vi "MemoryMapMain.vi"(8 "error in (no error)":errorcluster, 11 "MemoryMap in":refnum<class "MemoryMap.lvclass">) -> (3 "MemoryMap out":refnum<class "MemoryMap.lvclass">)   [LabVIEW 2020, in "Sgraph_lib_V1.lvlib" / "MemoryMap.lvclass"]
uses:
  MemoryMap.lvclass
  Gserver/controls/Typedef_Gviewer-Query.ctl
  Gserver/controls/Typedef_QueryType.ctl
  Common/controls/MeMapInfo.ctl
  Common/controls/MMap_element.ctl
  <vilib>/Utility/miscctls.llb/LVPoint32TypeDef.ctl
  Builds/Sgraph_lib_V1.lvlib
  Gserver/Gserver.lvclass
panel:
  in  "Layer":i32 min=0 max=6
  out "Graph 3":cluster{"Array":dbl[]}[](graph)
  out "Graph 2":cluster{"Array":dbl[]}[](graph)
  out "Graph 1":cluster{"Array":dbl[]}[](graph)
  out "37x37":picture
  in  "Gserver-Queue":refnum<queue>
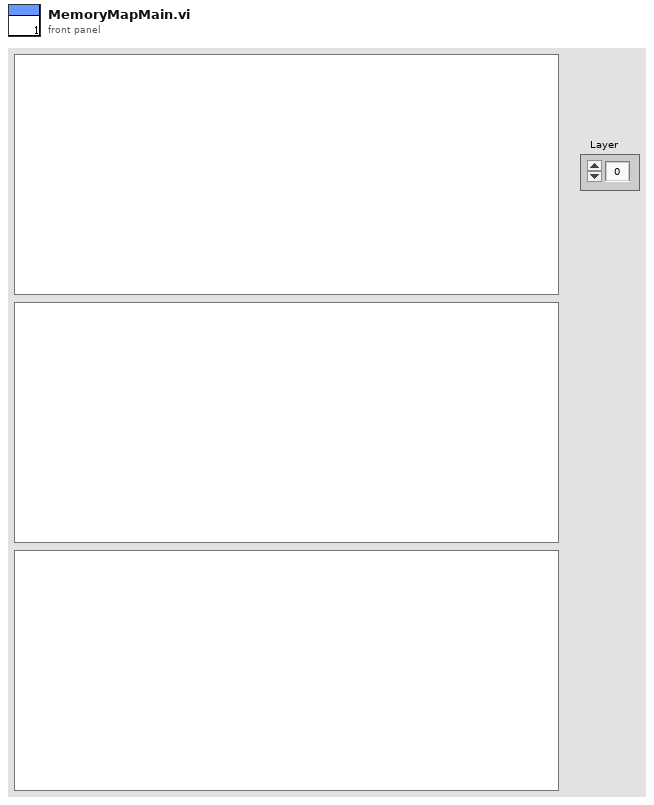
[diagram p1: front panel]
types:
  T1 = typedef "Sgraph_lib_V1.lvlib/MeMapInfo.ctl" = cluster{"MemLayer":T2[]}
  T2 = typedef "Sgraph_lib_V1.lvlib/MMap_element.ctl" = cluster{"Name":string, "Length":i32, "Pointer":i32, "Tbegin":dbl, "Tend":dbl, "Tmin":dbl, "Tmax":dbl, "Tpnt-1":dbl, "Tpnt":dbl, "Tpnt+1":dbl, "Array":dbl[]}
  T3 = typedef "LVBoundsTypeDef.ctl" = cluster{"Width":u32, "Height":u32}
  T4 = typedef "Sgraph_lib_V1.lvlib/Gserver.lvclass/Typedef_QueryType.ctl" = enum16{"Subscribe", "DataRequest", "RequestAllTags", "RequestIniPath", "FAMMstarted", "SetClientOptions", "GviewerUpdate", "OpenNewGraph", "CloseClient", "CloseAllClients", "Close Gserver", "OpenMemoryMap", "MeMapDataRequest", "MeMapDataResponse", "OpenDBeditor", "CheckDBeditorRunning", "StoppedDBeditor", "SaveDB_TAGpropRecord", "ConfirmDB_TAGpropSave"}
  T5 = typedef "Sgraph_lib_V1.lvlib/Gserver.lvclass/Typedef_Gviewer-Query.ctl" = cluster{"Query_type":T4, "data":variant, "Source":string, "Time Stamp":timestamp}
  T6 = cluster{"horizontal":enum16{"left", "center", "right"}, "vertical":enum16{"top", "center", "bottom"}}
  T7 = typedef "LVPoint32TypeDef.ctl" = cluster{"Horizontal":i32, "Vertical":i32}
  T8 = typedef "LVRectTypeDef.ctl" = cluster{"Left":i16, "Top":i16, "Right":i16, "Bottom":i16}
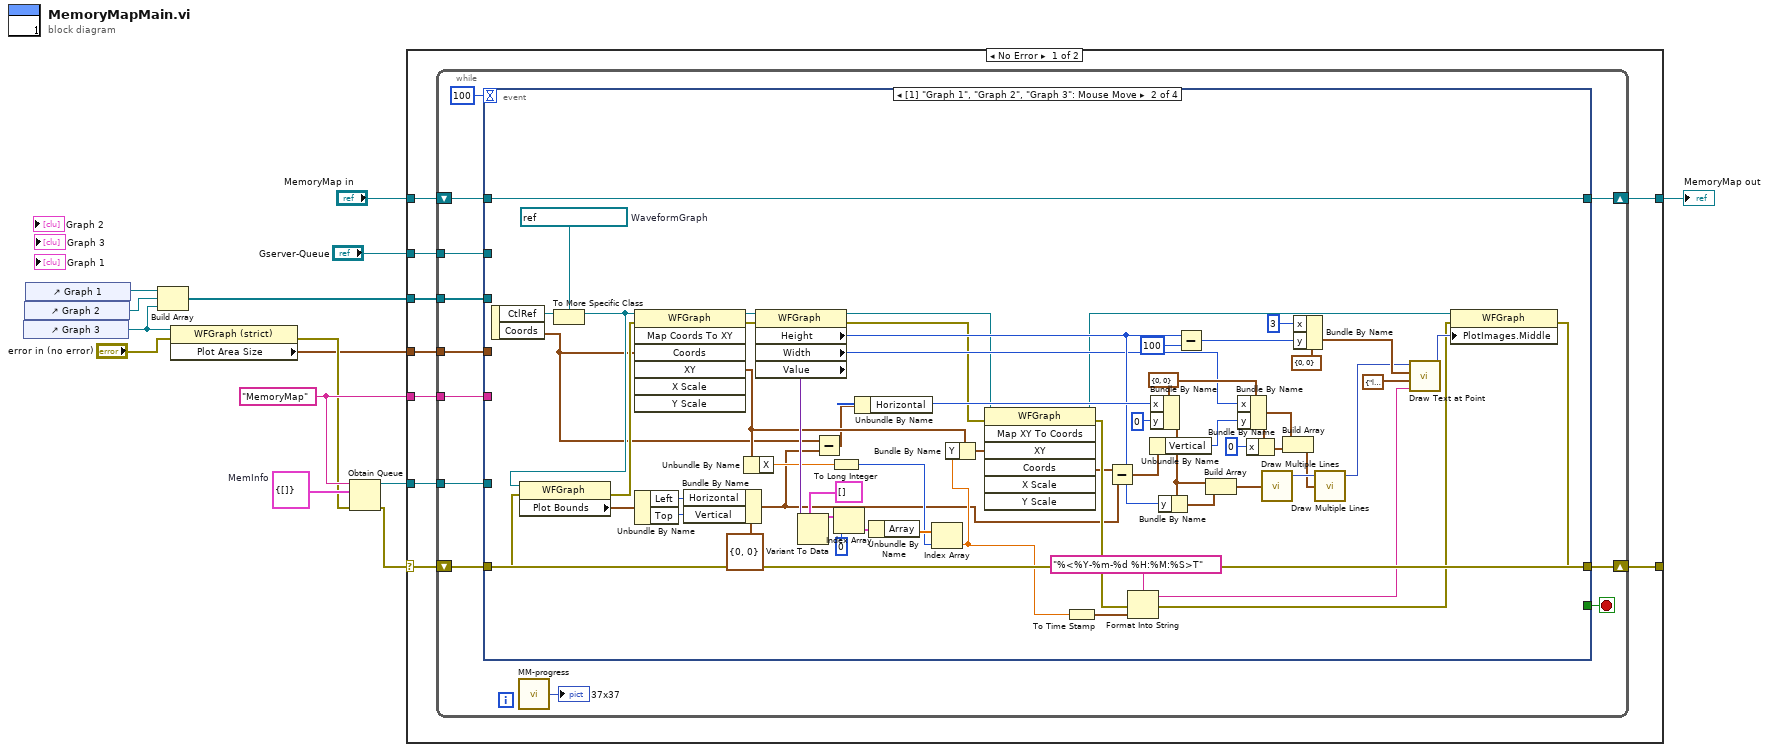
[diagram p0: block diagram]
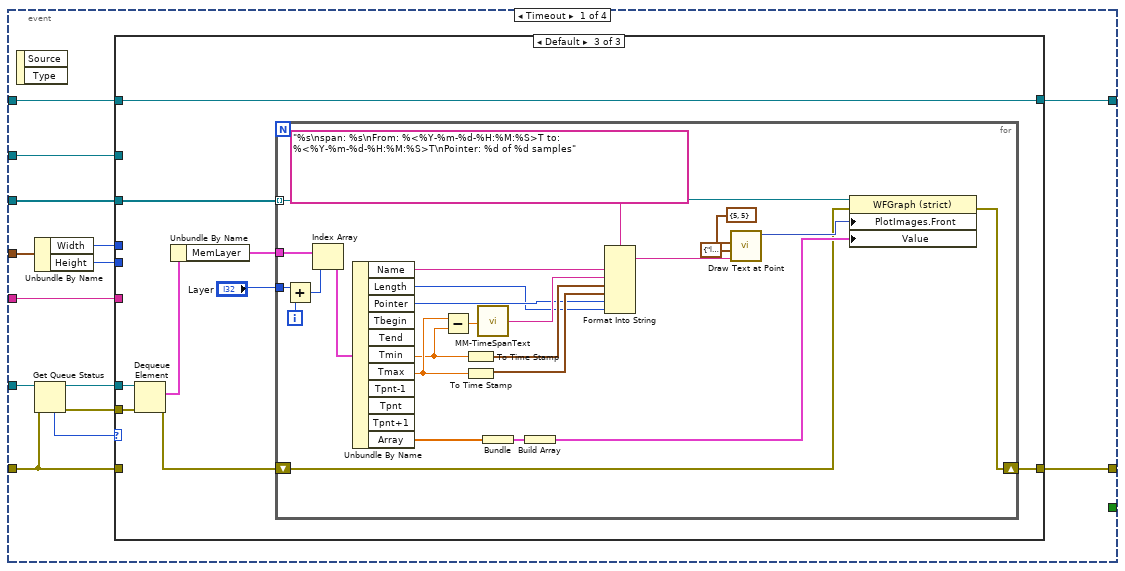
[diagram p2: hidden frame]
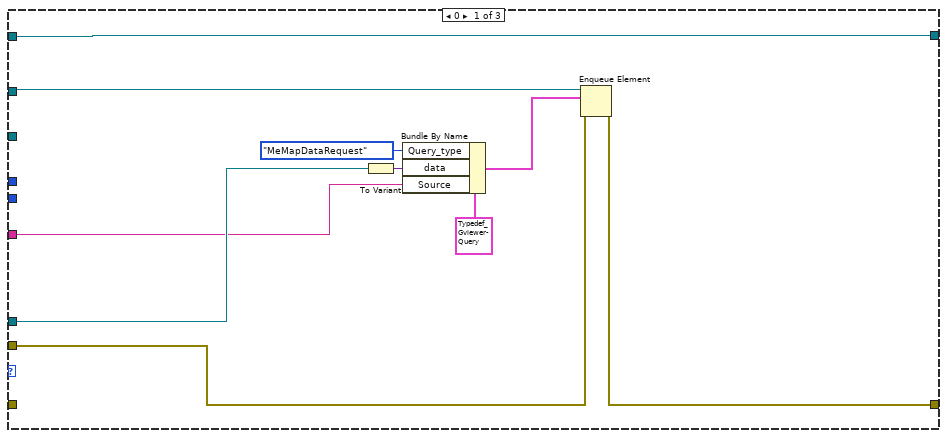
[diagram p3: hidden frame]
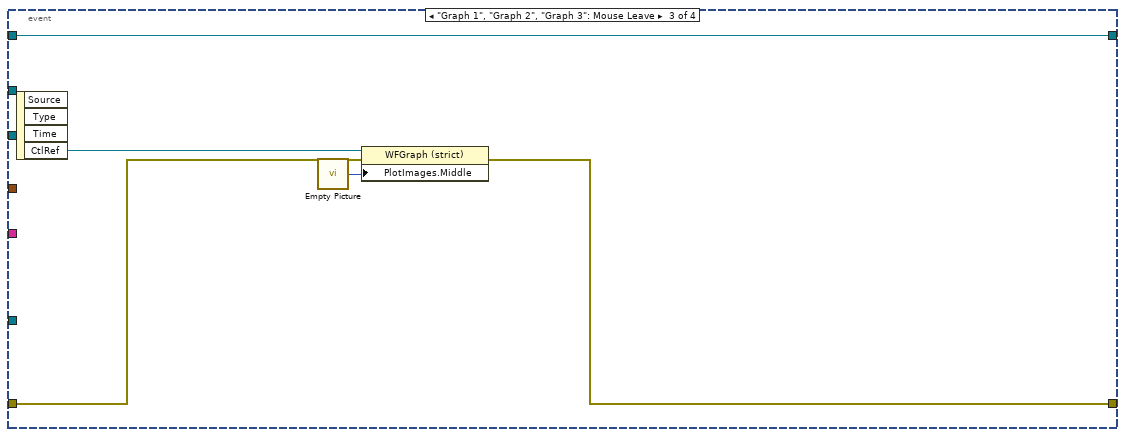
[diagram p5: hidden frame]
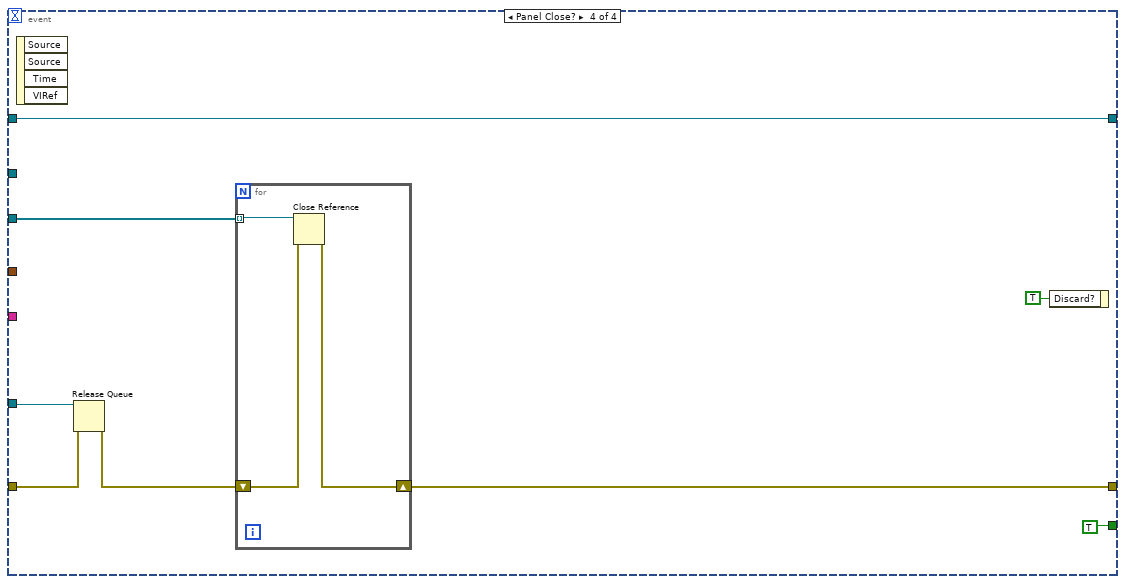
[diagram p6: hidden frame]
diagram:
  w8 = "MemoryMap" ("name (unnamed)")
  w11 = T1 {"MemLayer"=[]}  # MemInfo
  n1 = control-ref of="Graph 3"() -> (w4:refnum<vi>)
  n2 = control-ref of="Graph 2"() -> (w5:refnum<vi>)
  n3 = control-ref of="Graph 1"() -> (w6:refnum<vi>)
  n4 = Build Array(w6, w5, w4) -> (w7:refnum<vi>[])
  n5 = property class="WFGraph (strict)"(reference=w4, error in="error in (no error)") -> (error out=w2:errorcluster, "Plot Area Size"=w1:T3)  [unwired: 1 out]
  n6 = Obtain Queue(name (unnamed)=w8, element data type=w11, error in (no error)=w2) -> (queue out=w9:refnum<queue>, error out=w10:errorcluster)  [unwired: 2 in, 1 out]
  n7 = case shown="No Error" w10 {
    selector: w10 -> [w21 w170]
    tunnel: [w21 w170] -> _
    tunnel: [w20 w169] -> w13
    tunnel: "MemoryMap in" -> [w20 w169]
    tunnel: "Gserver-Queue" -> [w19 _]
    tunnel: w9 -> [w18 _]
    tunnel: w8 -> [w17 _]
    tunnel: w7 -> [w16 _]
    tunnel: w1 -> [w15 _]
    frame No Error {
      n8 = while {
        shift-right: [w30] -> _
        shift-left: w20 -> [w32]
        shift-right: [w29] -> _
        shift-left: w21 -> [w31]
        tunnel: w19 -> [w28]
        tunnel: w18 -> [w27]
        tunnel: w17 -> [w26]
        tunnel: w16 -> [w25]
        tunnel: w15 -> [w22]
        stop <- w23 stop-if-true
        n9 = event shown="[1] \"Graph 1\", \"Graph 2\", \"Graph 3\": Mouse Move" {
          selector: _ -> [_ _ _ _]
          dyn-events: _ -> [_ _ _ _]
          timeout: 100 -> [_ _ _ _]
          tunnel: w32 -> [w47 w126 w155 w163]
          tunnel: w31 -> [w34 w107 w154 w161]
          tunnel: [w46 w126 w155 w163] -> w30
          tunnel: [w45 w94 w156 w159] -> w29
          tunnel: w28 -> [w36 _ _ _]
          tunnel: w27 -> [w44 _ _ w162]
          tunnel: w26 -> [w35 _ _ _]
          tunnel: w25 -> [w43 _ _ w158]
          tunnel: [_ _ _ TRUE] -> w23
          tunnel: w22 -> [w39 _ _ _]
          event Timeout {
            n10 = event-data() -> ()  [unwired: 1 in, 2 out]
            n11 = Unbundle By Name(w39) -> ("Width"=w38:u32, "Height"=w37:u32)
            n12 = Get Queue Status(queue=w44, error in (no error)=w34) -> (queue out=w40:refnum<queue>, error out=w41:errorcluster, # elements in queue=w42:i32)  [unwired: 1 in, 5 out]
            n13 = case shown="Default" w42 {
              tunnel: w47 -> [w57 w58 w68]
              tunnel: [w57 w58 w68] -> w46
              tunnel: w41 -> [w48 _ w66]
              tunnel: [w49 w59 w61] -> w45
              tunnel: w40 -> [w53 _ w67]
              tunnel: w43 -> [_ _ w63]
              tunnel: w38 -> [_ _ _]
              tunnel: w37 -> [_ _ _]
              tunnel: w36 -> [w56 _ _]
              tunnel: w35 -> [w51 _ _]
              tunnel: w34 -> [_ w59 _]
              frame 0 {
                n14 = To Variant(anything=w53) -> (Variant=w52:variant)
                n15 = Bundle By Name(cluster=T5 {"Query_type"=enum."MeMapDataRequest", "data"=variant, "Source"="", "Time Stamp"=timestamp(0 s since 1904-01-01)} ("element"), "Query_type"=Typedef_QueryType."MeMapDataRequest", "data"=w52, "Source"=w51) -> (w50:T5)
                n16 = Enqueue Element(queue=w56, element=w50, error in (no error)=w48) -> (error out=w49:errorcluster)  [unwired: 1 in, 2 out]
              }
              frame -1 {
              }
              frame Default {
                n17 = Dequeue Element(queue=w67, error in (no error)=w66) -> (element=w65:T1, error out=w62:errorcluster)  [unwired: 1 in, 2 out]
                n18 = Unbundle By Name(w65) -> ("MemLayer"=w64:T2[])
                n19 = for {
                  tunnel: w64 -> [w84]
                  tunnel: w63 -> [w85] mode=indexing
                  shift-right: [w86] -> w61
                  shift-left: w62 -> [w87]
                  tunnel: "Layer" -> [w73]
                  i -> [w72]
                  n20 = Add(x=w73, y=w72) -> (x+y=w71:i32)
                  n21 = Index Array(array=w84, index=w71) -> (element=w83:T2)
                  n22 = Unbundle By Name(w83) -> ("Name"=w82:string, "Length"=w69:i32, "Pointer"=w70:i32, "Tmin"=w74:dbl, "Tmax"=w79:dbl, "Array"=w93:dbl[])  [unwired: 5 out]
                  n23 = Subtract(x=w79, y=w74) -> (x-y=w78:dbl)
                  n24 = To Time Stamp(1:w74) -> (0:w76:timestamp)
                  n25 = To Time Stamp(1:w79) -> (0:w75:timestamp)
                  n26 = call "MM-TimeSpanText.vi"("Timespan"=w78) -> ("TimeSpanText"=w77:string)  [unwired: 4 in]
                  n27 = Bundle("Array"=w93) -> (w89:cluster{"Array":dbl[]})  [unwired: 1 in]
                  n28 = Build Array(w89) -> (w88:cluster{"Array":dbl[]}[])
                  n29 = Format Into String(format string="%s\nspan: %s\nFrom: %<%Y-%m-%d-%H:%M:%S>T to: %<%Y-%m-%d-%H:%M:%S>T\nPointer: %d of %d samples", w82, w77, w76, w75, w70, w69) -> (resulting string=w81:string)  [unwired: 2 in, 1 out]
                  n30 = call <vilib>:"Draw Text at Point.vi"("text"=w81, "alignment(left, top)"=T6 {"horizontal"=enum."left", "vertical"=enum."top"}, "origin"=cluster{"x":i16, "y":i16} {"x"=5, "y"=5}) -> ("new picture"=w90:picture)  [unwired: 7 in, 1 out]
                  n31 = property class="WFGraph (strict)"(reference=w85, error in=w87, "PlotImages.Front"=w90, "Value"=w88) -> (error out=w86:errorcluster)  [unwired: 1 out]
                }
              }
            }
          }
          event "Graph 1", "Graph 2", "Graph 3": Mouse Move {
            w133 = cluster{"x":i16, "y":i16} {"x"=0, "y"=0}
            w152 = refnum<vi> refnum  # WaveformGraph
            n32 = event-data() -> ("CtlRef"=w109:refnum<vi>, "Coords"=w99:T7)  [unwired: 1 in]
            n33 = To More Specific Class(target class=w152, reference=w109) -> (specific class reference=w108:refnum<vi>)  [unwired: 1 in, 1 out]
            n34 = property class="WFGraph"(reference=w108, error in=w107) -> (error out=w106:errorcluster, "Plot Bounds"=w104:T8)  [unwired: 1 out]
            n35 = invoke class="WFGraph" method="Map Coords To XY"(reference=w108, error in=w106, "Coords"=w99) -> (reference out=w151:refnum<vi>, error out=w125:errorcluster, "XY"=w113:cluster{"X":dbl, "Y":dbl})  [unwired: 4 in, 4 out]
            n36 = Unbundle By Name(w104) -> ("Left"=w101:i16, "Top"=w102:i16)
            n37 = Bundle By Name(cluster=T7 {"Horizontal"=0, "Vertical"=0} ("Coords"), "Horizontal"=w101, "Vertical"=w102) -> (w97:T7)
            n38 = Unbundle By Name(w113) -> ("X"=w118:dbl)
            n39 = property class="WFGraph"(reference=w151, error in=w125) -> (reference out=w115:refnum<vi>, error out=w116:errorcluster, "Height"=w138:u32, "Width"=w131:u32, "Value"=w123:variant)
            n40 = Variant To Data(type=cluster{"Array":dbl[]}[] [] ("appended array"), Variant=w123) -> (data=w122:cluster{"Array":dbl[]}[])  [unwired: 1 in, 1 out]
            n41 = Subtract(x=w99, y=w97) -> (x-y=w100:T7)
            n42 = To Long Integer(number=w118) -> (32bit integer=w117:i32)
            n43 = Index Array(array=w122, index=0) -> (element=w120:cluster{"Array":dbl[]})
            n44 = Unbundle By Name(w100) -> ("Horizontal"=w147:i32)
            n45 = Unbundle By Name(w120) -> ("Array"=w119:dbl[])
            n46 = Index Array(array=w119, index=w117) -> (element=w111:dbl)
            n47 = Bundle By Name(cluster=w113, "Y"=w111) -> (w112:cluster{"X":dbl, "Y":dbl})
            n48 = invoke class="WFGraph" method="Map XY To Coords"(reference=w115, error in=w116, "XY"=w112) -> (reference out=w114:refnum<vi>, error out=w105:errorcluster, "Coords"=w98:T7)  [unwired: 4 in, 4 out]
            n49 = To Time Stamp(1:w111) -> (0:w145:timestamp)
            n50 = Subtract(x=w98, y=w97) -> (x-y=w96:T7)
            n51 = Format Into String(format string="%<%Y-%m-%d %H:%M:%S>T", error in=w105, w145) -> (resulting string=w142:string, error out=w95:errorcluster)  [unwired: 1 in]
            n52 = Unbundle By Name(w96) -> ("Vertical"=w110:i32)
            n53 = Bundle By Name(cluster=w133, "x"=w147, "y"=i16 0) -> (w141:cluster{"x":i16, "y":i16})
            n54 = Bundle By Name(cluster=w141, "y"=w138) -> (w149:cluster{"x":i16, "y":i16})
            n55 = Subtract(x=w138, y=100) -> (x-y=w137:u32)
            n56 = Build Array(w141, w149) -> (w148:cluster{"x":i16, "y":i16}[])
            n57 = Bundle By Name(cluster=w133, "x"=w131, "y"=w110) -> (w128:cluster{"x":i16, "y":i16})
            n58 = Bundle By Name(cluster=w128, "x"=i16 0) -> (w129:cluster{"x":i16, "y":i16})
            n59 = call <vilib>:"Draw Multiple Lines.vi"("line endpoints"=w148) -> ("new picture"=w135:picture)  [unwired: 8 in]
            n60 = Build Array(w128, w129) -> (w127:cluster{"x":i16, "y":i16}[])
            n61 = Bundle By Name(cluster=cluster{"x":i16, "y":i16} {"x"=0, "y"=0}, "x"=i16 3, "y"=w137) -> (w140:cluster{"x":i16, "y":i16})
            n62 = call <vilib>:"Draw Multiple Lines.vi"("picture"=w135, "line endpoints"=w127) -> ("new picture"=w134:picture)  [unwired: 7 in]
            n63 = call <vilib>:"Draw Text at Point.vi"("text"=w142, "alignment(left, top)"=T6 {"horizontal"=enum."left", "vertical"=enum."bottom"}, "origin"=w140, "picture"=w134) -> ("new picture"=w143:picture)  [unwired: 6 in, 1 out]
            n64 = property class="WFGraph"(reference=w114, error in=w95, "PlotImages.Middle"=w143) -> (error out=w94:errorcluster)  [unwired: 1 out]
          }
          event "Graph 1", "Graph 2", "Graph 3": Mouse Leave {
            n65 = event-data() -> ("CtlRef"=w157:refnum<vi>)  [unwired: 1 in, 3 out]
            n66 = call "Empty Picture"() -> ("empty picture"=w153:picture)
            n67 = property class="WFGraph (strict)"(reference=w157, error in=w154, "PlotImages.Middle"=w153) -> (error out=w156:errorcluster)  [unwired: 1 out]
          }
          event Panel Close? {
            n68 = event-data() -> ()  [unwired: 1 in, 4 out]
            n69 = Release Queue(queue=w162, error in (no error)=w161) -> (error out=w160:errorcluster)  [unwired: 1 in, 2 out]
            n70 = for {
              shift-right: [w166] -> w159
              shift-left: w160 -> [w167]
              tunnel: w158 -> [w168] mode=indexing
              n71 = Close Reference(reference=w168, error in (no error)=w167) -> (error out=w166:errorcluster)
            }
            n72 = event-data("Discard?"=TRUE) -> ()  [unwired: 1 in, 1 out]
          }
        }
        n73 = call "MM-progress.vi"() -> ("37x37"=→"37x37":picture)  [unwired: 7 in]
      }
    }
    frame Error {
    }
  }
  "MemoryMap out" <- w13
